vi "gfitsio-get-num-cols.vi"(8 "error in (no error)":errorcluster, 11 "gfits refnum":T1) -> (0 "error out":errorcluster, 2 "number of columns":i32, 3 "dup gfits refnum":T1)   [LabVIEW 2019, in "gfitsio.lvlib"]
doc: "Get the number of columns in the current FITS table."
uses:
  gfitsio.lvlib
  gfitsio-refnum.ctl
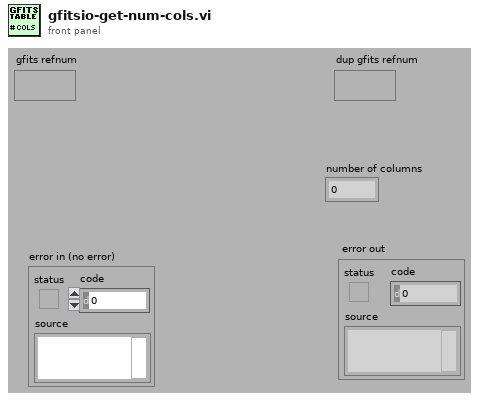
[diagram p1: front panel]
types:
  T1 = typedef "gfitsio.lvlib/gfitsio-refnum.ctl" = refnum<k1>
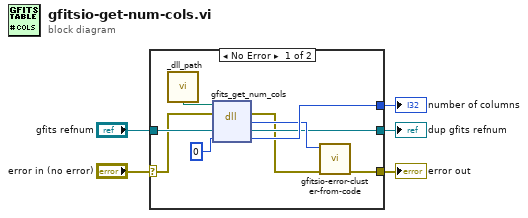
[diagram p0: block diagram]
diagram:
  n1 = case shown="No Error" "error in (no error)" {
    selector: "error in (no error)" -> [w8 w16]
    tunnel: [w12 w16] -> w5
    tunnel: "gfits refnum" -> [w10 w15]
    tunnel: [w11 w15] -> w3
    tunnel: [w14 _] -> w1
    frame No Error {
      n2 = call "_dll_path.vi"() -> ("Path"=w6:path)  [unwired: 1 in]
      n3 = dll-call lib="?" fn="gfits_get_num_cols"(path in=w6, error in=w8, "refnum"=w10, "nrows"=0) -> (error out=w7:errorcluster, "return type"=w13:i32, "refnum"=w11:T1, "nrows"=w14:i32)  [unwired: 1 in, 1 out]
      n4 = call "gfitsio-error-cluster-from-code.vi"("error in (no error)"=w7, "error code"=w13) -> ("error out"=w12:errorcluster)  [unwired: 9 out]
    }
    frame Error {
    }
  }
  "error out" <- w5
  "dup gfits refnum" <- w3
  "number of columns" <- w1
